vi "Jog.vi"(1 "Direction":string, 2 "Step Amount":dbl) -> (7 "Array":string[](array[string]))   [LabVIEW 2021]
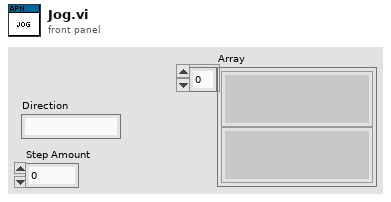
[diagram p1: front panel]
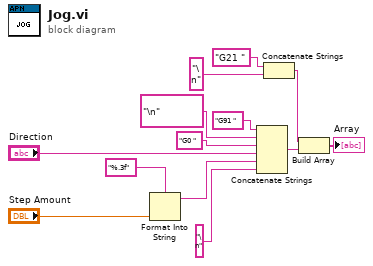
[diagram p0: block diagram]
diagram:
  n1 = Format Into String(format string="%.3f", "Step Amount") -> (resulting string=w8:string)  [unwired: 2 in, 1 out]
  n2 = Concatenate Strings("G91 " ("string"), "\n" ("string"), "G0 " ("string"), "Direction", w8, "\n" ("string")) -> (w6:string)
  n3 = Concatenate Strings("G21 ", "\n" ("string")) -> (w7:string)
  n4 = Build Array(w7, w6) -> (→"Array":string[])
